vi "GV_Bypass_Global.vi"() -> ()   [LabVIEW 2019]
panel:
  out "GVB_ST":u32(colorbox)
  out "GVB_turn":dbl
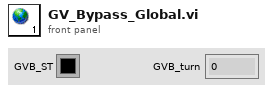
[diagram p1: front panel]
diagram:
